vi "ke37xx Initiate Scan on Totalizer Match.vi"() -> ()   [LabVIEW 2009]
uses:
  <instrlib>/Keithley 3706/Keithley 3700 Series.lvlib
panel:
  in  "Pseudocard Slot":u8=1 min=1 max=6
  out "Scan State":string
  out "Totalizer Count Display":u32(slide) scale=0.0..1000.0
  out "Match Detected":bool
  in  "Totalizer Channel":string
  in  "Value to Match":u32
  out "error out":errorcluster
  in  "VISA Resource Name":refnum<visa-resource-name>
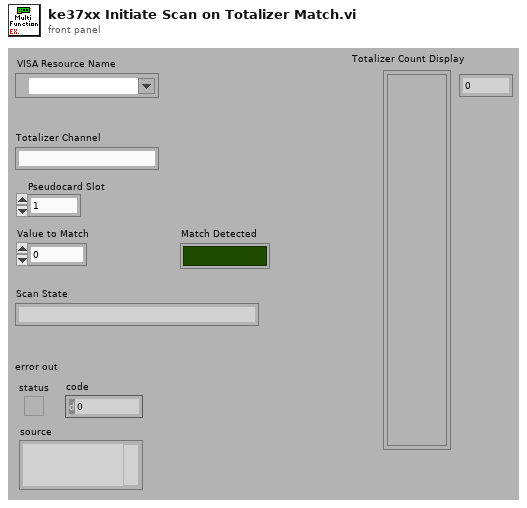
[diagram p1: front panel]
types:
  T1 = enum16{"Empty", "Building", "Running", "Aborted", "Failed", "Failed Init", "Success"}
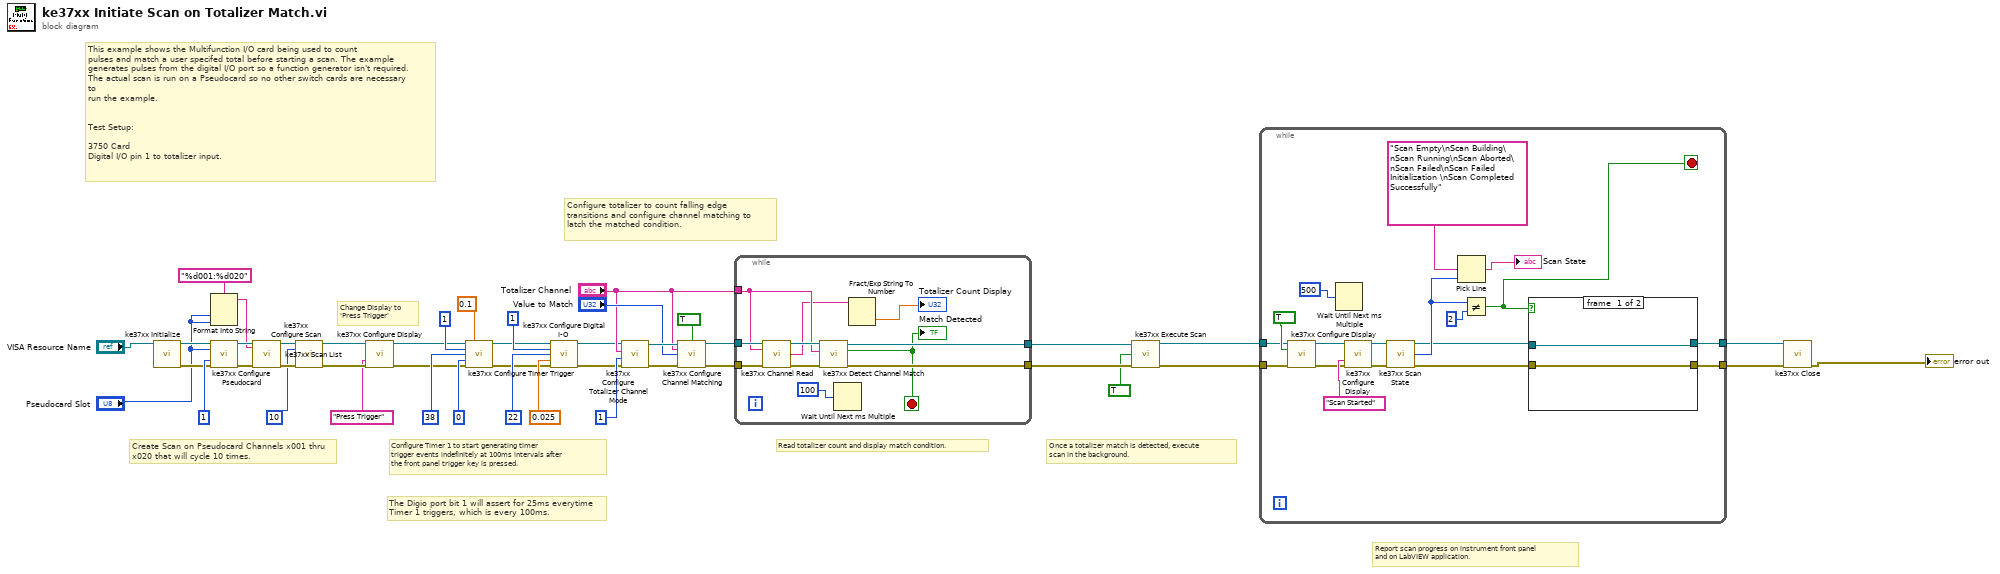
[diagram p0: block diagram]
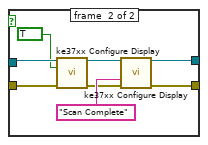
[diagram p2: hidden frame]
diagram:
  # "Read totalizer count and display match condition."
  # "Report scan progress on instrument front panel\nand on LabVIEW application."
  # "Once a totalizer match is detected, execute\nscan in the background."
  # "This example shows the Multifunction I/O card being used to count\npulses and match a user specifed total before starting a scan. The example\ngenerates pulses from the digital I/O port so a function generator isn't required.\nThe actual scan is run on a Pseudocard so no other switch cards are necessary to\nrun the example. \n\n\nTest Setup:\n\n3750 Card\nDigital I/O pin 1 to totalizer input."
  # "Change Display to\n'Press Trigger'"
  # "The Digio port bit 1 will assert for 25ms everytime\nTimer 1 triggers, which is every 100ms."
  # "Configure Timer 1 to start generating timer\ntrigger events indefinitely at 100ms intervals after\nthe front panel trigger key is pressed."
  # "Create Scan on Pseudocard Channels x001 thru\nx020 that will cycle 10 times."
  # "Configure totalizer to count falling edge transitions and configure channel matching to latch the matched condition."
  n1 = call <instrlib>:"ke37xx Initialize.vi"("VISA resource name"="VISA Resource Name") -> ("VISA resource name out"=w16:refnum<visa-resource-name>, "error out"=w15:errorcluster)  [unwired: 13 in]
  n2 = Format Into String(format string="%d001:%d020", "Pseudocard Slot", "Pseudocard Slot") -> (resulting string=w4:string)  [unwired: 2 in, 1 out]
  n3 = call <instrlib>:"ke37xx Configure Pseudocard.vi"("VISA Resource Name"=w16, "Slot Number (1)"="Pseudocard Slot", "Pseudocard Name (1: 3720)"=1, "error in (no error)"=w15) -> ("VISA Resource Name Out"=w38:refnum<visa-resource-name>, "error out"=w37:errorcluster)  [unwired: 10 in]
  n4 = call <instrlib>:"ke37xx Scan List.vi"("VISA Resource Name"=w38, "Channel List"=w4, "error in (no error)"=w37) -> ("VISA Resource Name Out"=w36:refnum<visa-resource-name>, "error out"=w35:errorcluster)  [unwired: 10 in, 1 out]
  n5 = call <instrlib>:"ke37xx Configure Scan.vi"("VISA Resource Name"=w36, "Scan Count (1)"=10, "error in (no error)"=w35) -> ("VISA Resource Name Out"=w27:refnum<visa-resource-name>, "error out"=w26:errorcluster)  [unwired: 11 in]
  n6 = call <instrlib>:"ke37xx Configure Display.vi"("VISA Resource Name"=w27, "Message (Empty)"="Press Trigger", "error in (no error)"=w26) -> ("VISA Resource Name Out"=w24:refnum<visa-resource-name>, "error out"=w23:errorcluster)  [unwired: 11 in]
  n7 = call <instrlib>:"ke37xx Configure Timer Trigger.vi"("VISA Resource Name"=w24, "Delay (1E-5 sec)"=0.1, "Timer (1)"=1, "Stimulus (0: None)"=38, "Count (1)"=0, "error in (no error)"=w23) -> ("VISA Resource Name Out"=w22:refnum<visa-resource-name>, "error out"=w21:errorcluster)  [unwired: 8 in]
  n8 = call <instrlib>:"ke37xx Configure Digital I-O.vi"("VISA Resource Name"=w22, "Line (1)"=1, "Stimulus (0: None)"=22, "Pulse Width (10 sec)"=0.025, "error in (no error)"=w21) -> ("VISA Resource Name Out"=w10:refnum<visa-resource-name>, "error out"=w9:errorcluster)  [unwired: 9 in]
  n9 = call <instrlib>:"ke37xx Configure Totalizer Channel Mode.vi"("error in (no error)"=w9, "Mode (Rising Edge TTL)"=1, "Totalizer Channels"="Totalizer Channel", "VISA Resource Name"=w10) -> ("error out"=w42:errorcluster, "VISA Resource Name Out"=w41:refnum<visa-resource-name>)  [unwired: 6 in]
  n10 = call <instrlib>:"ke37xx Configure Channel Matching.vi"("VISA Resource Name"=w41, "Match State Latching (True)"=TRUE, "Specified Channels"="Totalizer Channel", "Match Value"="Value to Match", "error in (no error)"=w42) -> ("VISA Resource Name Out"=w20:refnum<visa-resource-name>, "error out"=w19:errorcluster)  [unwired: 9 in]
  n11 = while {
    tunnel: w20 -> [w49]
    tunnel: w19 -> [w50]
    tunnel: "Totalizer Channel" -> [w48]
    tunnel: [w54] -> w18
    tunnel: [w53] -> w17
    stop <- w47 stop-if-true
    n12 = call <instrlib>:"ke37xx Channel Read.vi"("VISA Resource Name"=w49, "Channel"=w48, "error in (no error)"=w50) -> ("VISA Resource Name Out"=w52:refnum<visa-resource-name>, "Data Output"=w46:string, "error out"=w51:errorcluster)  [unwired: 10 in]
    n13 = call <instrlib>:"ke37xx Detect Channel Match.vi"("error in (no error)"=w51, "Channel to Check for Match"=w48, "VISA Resource Name"=w52) -> ("error out"=w53:errorcluster, "Matched"=w47:bool, "VISA Resource Name Out"=w54:refnum<visa-resource-name>)  [unwired: 6 in]
    "Match Detected" <- w47
    n14 = Wait Until Next ms Multiple(millisecond multiple=100) -> ()  [unwired: 1 out]
    n15 = Fract/Exp String To Number(string=w46) -> (number=→"Totalizer Count Display":dbl)  [unwired: 3 in, 1 out]
  }
  n16 = call <instrlib>:"ke37xx Execute Scan.vi"("VISA Resource Name"=w18, "Background (False)"=TRUE, "error in (no error)"=w17) -> ("VISA Resource Name Out"=w8:refnum<visa-resource-name>, "error out"=w7:errorcluster)  [unwired: 11 in]
  n17 = while {
    tunnel: w8 -> [w60]
    tunnel: w7 -> [w59]
    tunnel: [w63] -> w3
    tunnel: [w56] -> w2
    stop <- w62 stop-if-true
    n18 = call <instrlib>:"ke37xx Configure Display.vi"("VISA Resource Name"=w60, "Clear Display (False)"=TRUE, "error in (no error)"=w59) -> ("VISA Resource Name Out"=w57:refnum<visa-resource-name>, "error out"=w58:errorcluster)  [unwired: 11 in]
    n19 = Wait Until Next ms Multiple(millisecond multiple=500) -> ()  [unwired: 1 out]
    n20 = call <instrlib>:"ke37xx Configure Display.vi"("VISA Resource Name"=w57, "Message (Empty)"="Scan Started", "error in (no error)"=w58) -> ("VISA Resource Name Out"=w72:refnum<visa-resource-name>, "error out"=w71:errorcluster)  [unwired: 11 in]
    n21 = call <instrlib>:"ke37xx Scan State.vi"("VISA Resource Name"=w72, "error in (no error)"=w71) -> ("VISA Resource Name Out"=w65:refnum<visa-resource-name>, "Scan State"=w68:T1, "error out"=w64:errorcluster)  [unwired: 11 in]
    n22 = Pick Line(multi-line string="Scan Empty\nScan Building\nScan Running\nScan Aborted\nScan Failed\nScan Failed Initialization \nScan Completed Successfully", line index=w68) -> (output string=→"Scan State":string)  [unwired: 1 in]
    n23 = Not Equal?(x=w68, y=2) -> (x != y?=w62:bool)
    n24 = case shown="True" w62 {
      tunnel: w65 -> [w74 w81]
      tunnel: w64 -> [w75 w80]
      tunnel: [w75 w82] -> w63
      tunnel: [w74 w76] -> w56
      frame #0 {
      }
      frame #1 {
        n25 = call <instrlib>:"ke37xx Configure Display.vi"("VISA Resource Name"=w81, "Clear Display (False)"=TRUE, "error in (no error)"=w80) -> ("VISA Resource Name Out"=w79:refnum<visa-resource-name>, "error out"=w78:errorcluster)  [unwired: 11 in]
        n26 = call <instrlib>:"ke37xx Configure Display.vi"("VISA Resource Name"=w79, "Message (Empty)"="Scan Complete", "error in (no error)"=w78) -> ("VISA Resource Name Out"=w76:refnum<visa-resource-name>, "error out"=w82:errorcluster)  [unwired: 11 in]
      }
    }
  }
  n27 = call <instrlib>:"ke37xx Close.vi"("VISA resource name"=w2, "error in (no error)"=w3) -> ("error out"=→"error out":errorcluster)  [unwired: 13 in]
